vi "RunTest.vi"() -> ()   [LabVIEW 2016]
uses:
  main/apis/Setup/GetVI/GetVIByName.vi
  main/apis/Setup/GetVI/GetVIByPath.vi
  <vilib>/addons/_JKI Toolkits/Caraya/classes/Assert/Assert Not Error.vi
  DronaTest.lvlib
  main/Drona.lvlib
  main/apis/Setup/GetVI/GetVI.lvlib
  <vilib>/addons/_JKI Toolkits/Caraya/classes/Test/Test.lvclass
  <vilib>/addons/_JKI Toolkits/Caraya/classes/Assert/Assert.lvclass
panel:
  out "error out":errorcluster
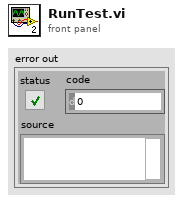
[diagram p1: front panel]
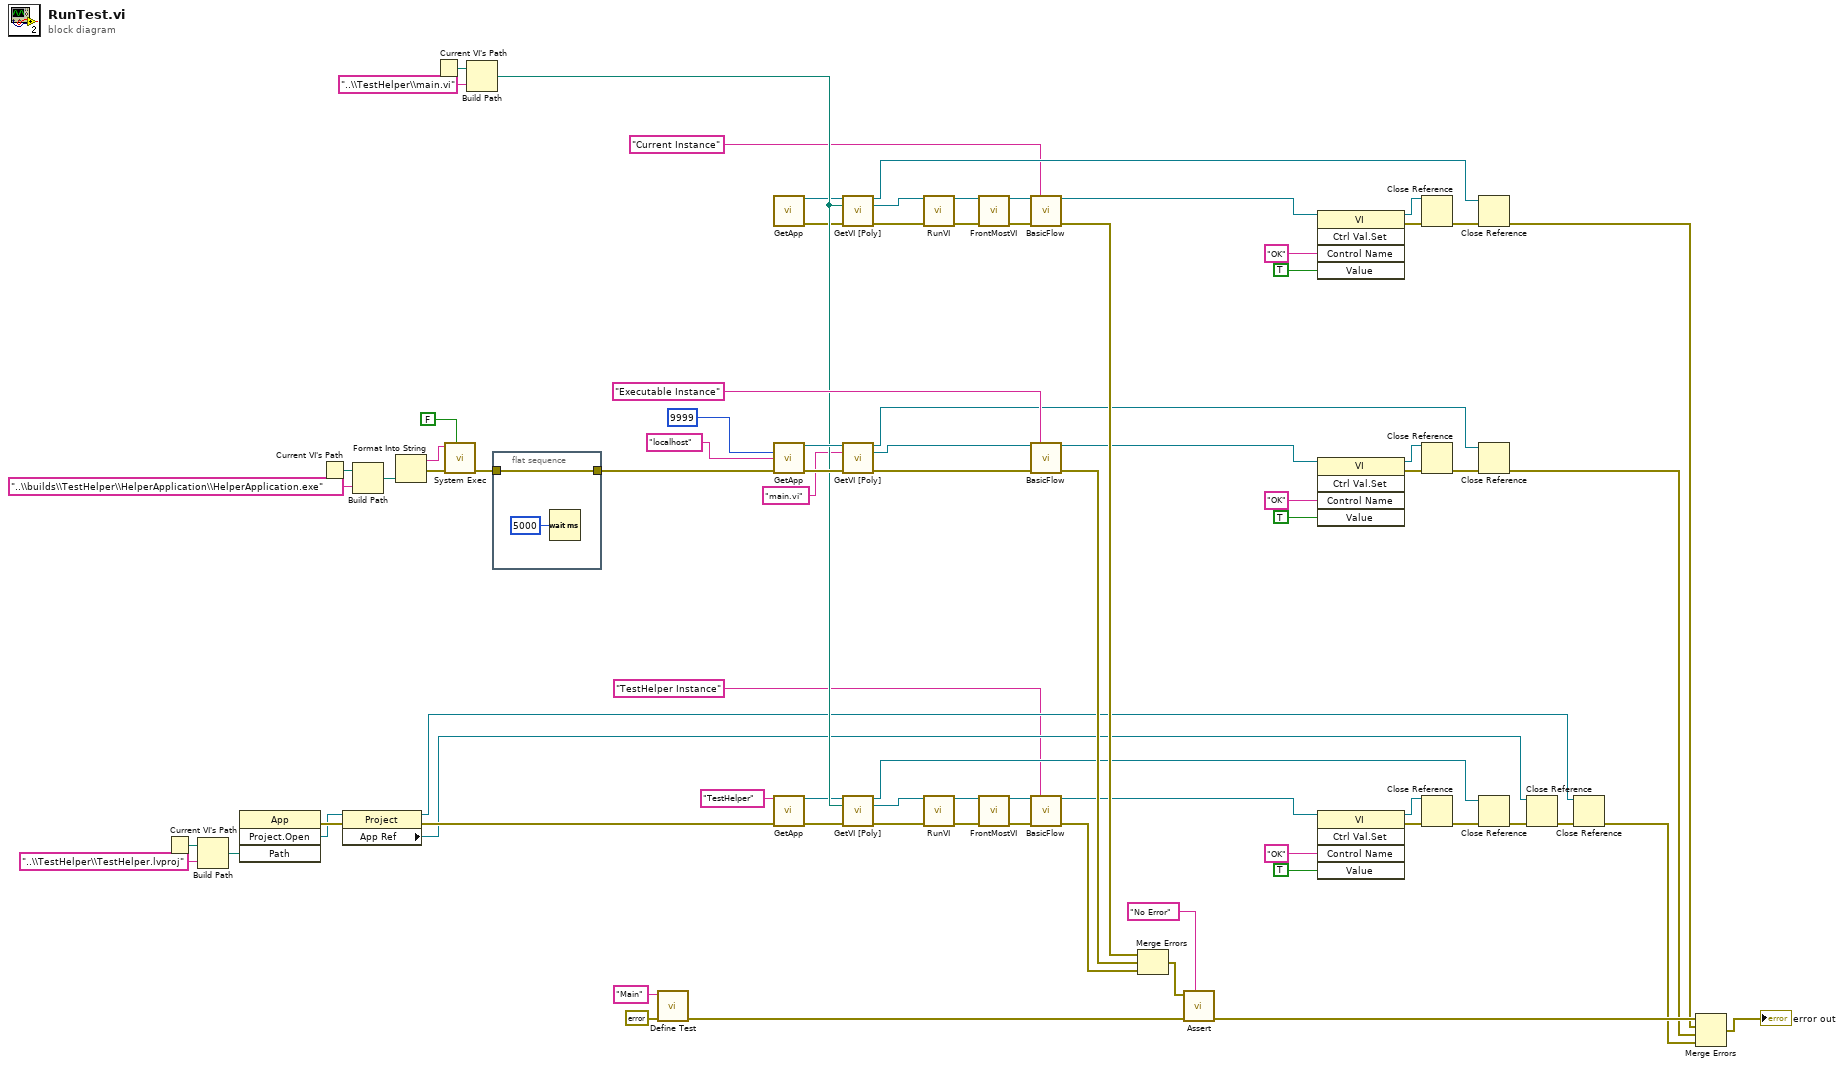
[diagram p0: block diagram]
diagram:
  n1 = Current VI's Path() -> (path=w17:path)
  n2 = Build Path(base path=w17, name or relative path="..\\TestHelper\\TestHelper.lvproj") -> (appended path=w15:path)
  n3 = invoke class="App" method="Project.Open"("Path"=w15) -> (error out=w19:errorcluster, "Project:Open"=w18:refnum<vi>)  [unwired: 3 in, 2 out]
  n4 = Current VI's Path() -> (path=w63:path)
  n5 = property class="Project"(reference=w18, error in=w19) -> (reference out=w13:refnum<vi>, error out=w14:errorcluster, "App Ref"=w12:refnum<vi>)
  n6 = Build Path(base path=w63, name or relative path="..\\builds\\TestHelper\\HelperApplication\\HelperApplication.exe") -> (appended path=w59:path)
  n7 = Format Into String(w59) -> (resulting string=w60:string, error out=w61:errorcluster)  [unwired: 3 in]
  n8 = Current VI's Path() -> (path=w43:path)
  n9 = call <vilib>:"System Exec.vi"("wait until completion? (T)"=FALSE, "error in (no error)"=w61, "command line"=w60) -> ("error out"=w46:errorcluster)  [unwired: 5 in, 3 out]
  n10 = Build Path(base path=w43, name or relative path="..\\TestHelper\\main.vi") -> (appended path=w67:path)
  n11 = flat-sequence {
    tunnel: [w84] -> w47
    tunnel: w46 -> [w84]
    frame #0 {
      n12 = Wait (ms)(milliseconds to wait=u32 5000) -> ()  [unwired: 1 out]
    }
  }
  n13 = call <vilib>:"Define Test.vi"("error in (no error)"=errorcluster {"status"=FALSE, "code"=0, "source"=""}, "Label (VI Title)"="Main") -> ("error out"=w78:errorcluster)  [unwired: 9 in]
  n14 = call "GetApp.vi"() -> ("Application Ref"=w44:refnum<vi>, "error out"=w45:errorcluster)  [unwired: 14 in]
  n15 = call "GetApp.vi"("Port(0:Ignored)"=u16 9999, "Service Name (\"\":localhost)"="localhost" ("Project Name (\"\": ThisApplication)"), "error in (no error)"=w47) -> ("Application Ref"=w69:refnum<vi>, "error out"=w68:errorcluster)  [unwired: 11 in]
  n16 = call "GetApp.vi"("Project Name (\"\": ThisApplication)"="TestHelper" ("Project Name (\"\": ThisApplication)"), "error in (no error)"=w14) -> ("Application Ref"=w21:refnum<vi>, "error out"=w20:errorcluster)  [unwired: 12 in]
  n17 = call-poly "GetVI [Poly].vi"("Application Ref in"=w44, "VI Path"=w67, "error in (no error)"=w45) -> ("Application Ref out"=w41:refnum<vi>, "VI Reference"=w40:refnum<vi>, "error out"=w39:errorcluster)  [unwired: 10 in]
  n18 = call-poly "GetVI [Poly].vi"("Application Ref in"=w69, "VI Name"="main.vi", "error in (no error)"=w68) -> ("Application Ref out"=w70:refnum<vi>, "VI Reference"=w48:refnum<vi>, "error out"=w71:errorcluster)  [unwired: 10 in]
  n19 = call-poly "GetVI [Poly].vi"("Application Ref in"=w21, "VI Path"=w67, "error in (no error)"=w20) -> ("Application Ref out"=w22:refnum<vi>, "VI Reference"=w23:refnum<vi>, "error out"=w24:errorcluster)  [unwired: 10 in]
  n20 = call "RunVI.vi"("VI Reference In"=w40, "error in"=w39) -> ("VI Reference Out"=w34:refnum<vi>, "error out"=w33:errorcluster)  [unwired: 12 in]
  n21 = call "RunVI.vi"("VI Reference In"=w23, "error in"=w24) -> ("VI Reference Out"=w9:refnum<vi>, "error out"=w8:errorcluster)  [unwired: 12 in]
  n22 = call "FrontMostVI.vi"("VI Reference In"=w34, "error in"=w33) -> ("VI Reference Out"=w37:refnum<vi>, "error out"=w38:errorcluster)  [unwired: 12 in]
  n23 = call "FrontMostVI.vi"("VI Reference In"=w9, "error in"=w8) -> ("VI Reference Out"=w26:refnum<vi>, "error out"=w25:errorcluster)  [unwired: 12 in]
  n24 = call "BasicFlow.vi"("VI Reference In"=w37, "Label (VI Title)"="Current Instance", "error in (no error)"=w38) -> ("VI Reference Out"=w36:refnum<vi>, "error out"=w76:errorcluster)  [unwired: 11 in]
  n25 = call "BasicFlow.vi"("VI Reference In"=w48, "Label (VI Title)"="Executable Instance", "error in (no error)"=w71) -> ("VI Reference Out"=w72:refnum<vi>, "error out"=w65:errorcluster)  [unwired: 11 in]
  n26 = call "BasicFlow.vi"("VI Reference In"=w26, "Label (VI Title)"="TestHelper Instance", "error in (no error)"=w25) -> ("VI Reference Out"=w27:refnum<vi>, "error out"=w74:errorcluster)  [unwired: 11 in]
  n27 = Merge Errors(w76, w65, w74) -> (w75:errorcluster)
  n28 = call-poly <vilib>:"Assert.vi"("Label"="No Error" ("Label (VI Title)"), "error in (no error)"=w78, "Not Error?"=w75) -> ("error out"=w81:errorcluster)  [unwired: 8 in]
  n29 = invoke class="VI" method="Ctrl Val.Set"(reference=w36, "Control Name"="OK", "Value"=TRUE) -> (reference out=w29:refnum<vi>, error out=w28:errorcluster)  [unwired: 2 in, 3 out]
  n30 = invoke class="VI" method="Ctrl Val.Set"(reference=w72, "Control Name"="OK", "Value"=TRUE) -> (reference out=w54:refnum<vi>, error out=w55:errorcluster)  [unwired: 2 in, 3 out]
  n31 = invoke class="VI" method="Ctrl Val.Set"(reference=w27, "Control Name"="OK", "Value"=TRUE) -> (reference out=w6:refnum<vi>, error out=w7:errorcluster)  [unwired: 2 in, 3 out]
  n32 = Close Reference(reference=w29, error in (no error)=w28) -> (error out=w32:errorcluster)
  n33 = Close Reference(reference=w54, error in (no error)=w55) -> (error out=w51:errorcluster)
  n34 = Close Reference(reference=w6, error in (no error)=w7) -> (error out=w3:errorcluster)
  n35 = Close Reference(reference=w41, error in (no error)=w32) -> (error out=w57:errorcluster)
  n36 = Close Reference(reference=w70, error in (no error)=w51) -> (error out=w50:errorcluster)
  n37 = Close Reference(reference=w22, error in (no error)=w3) -> (error out=w1:errorcluster)
  n38 = Close Reference(reference=w12, error in (no error)=w1) -> (error out=w2:errorcluster)
  n39 = Close Reference(reference=w13, error in (no error)=w2) -> (error out=w56:errorcluster)
  n40 = Merge Errors(w81, w57, w50, w56) -> (→"error out":errorcluster)
